vi "conversor.vi"(1 "Temperatura (C)":dbl(slide) scale=0.0..100.0) -> (0 "Temperatura (F)":dbl)   [LabVIEW 2020]
doc: "Converte de graus celsius para graus fahrenheit."
panel:
  # "Conversão de graus celsius para graus fahrenheit"
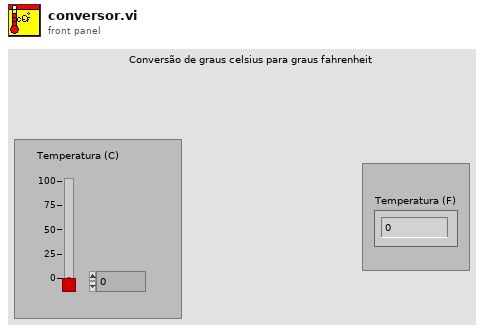
[diagram p1: front panel]
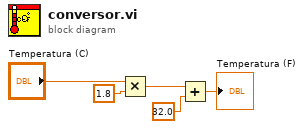
[diagram p0: block diagram]
diagram:
  n1 = Multiply(x="Temperatura (C)", y=1.8) -> (x*y=w3:dbl)
  n2 = Add(x=w3, y=32.0) -> (x+y=→"Temperatura (F)":dbl)
